vi "Test Array.vi"(10 "Index":dbl, 11 "Array":dbl[](array[numeric]) caption="Array2") -> (3 "Gauge":dbl(knob) scale=0.0..10.0)   [LabVIEW 2024]
doc: "This is Test 3 vi."
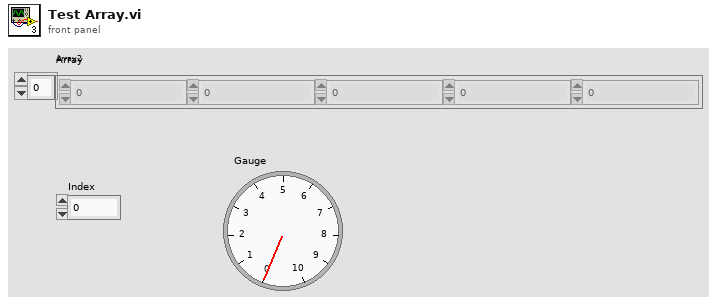
[diagram p1: front panel]
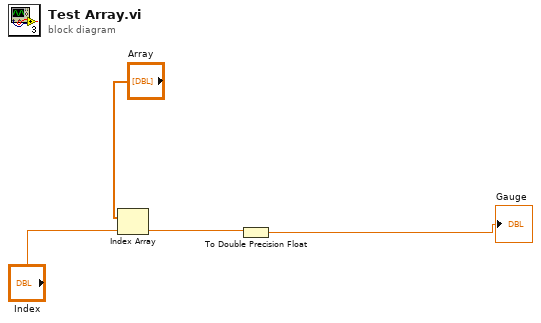
[diagram p0: block diagram]
diagram:
  n1 = Index Array(array="Array", index="Index") -> (element=w2:dbl)
  n2 = To Double Precision Float(number=w2) -> (double precision float=→"Gauge":dbl)
